vi "OFDM_SuperpositionedBitDetect.vi"(0 "Input symbols":cdb[](array[numeric]) format="%.2f", 1 "Modulation type":enum16{"QPSK(4QAM)", "64QAM", "16QAM", "BPSK"}(ring), 3 "error in (no error)":errorcluster) -> (5 "Base Bits":i8[](array[numeric]), 7 "SC Bits":i8[](array[numeric]), 10 "error out":errorcluster)   [LabVIEW 2022 SP3]
uses:
  <vilib>/addons/Modulation/Digital/General/MT Map QAM Symbols to Bits.vi
  <vilib>/addons/Modulation/Digital/General/MT Map Bits to QAM Symbols.vi
  <vilib>/addons/Modulation/Digital/General/MT Map PSK Symbols to Bits.vi
  <vilib>/addons/Modulation/Digital/General/MT Map Bits to PSK Symbols.vi
  <vilib>/addons/Modulation/niDMT.lvlib
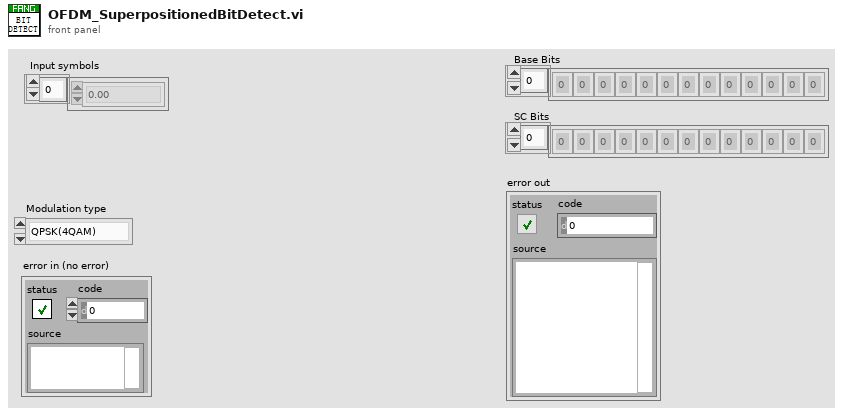
[diagram p1: front panel]
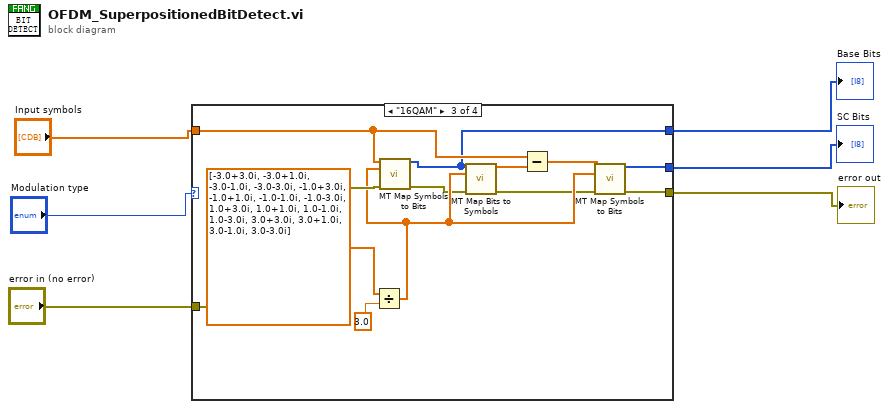
[diagram p0: block diagram]
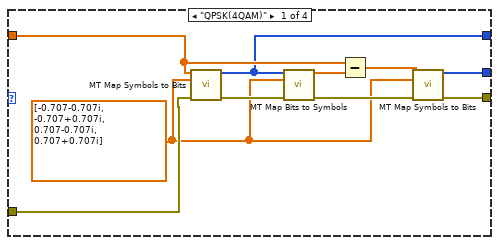
[diagram p2: hidden frame]
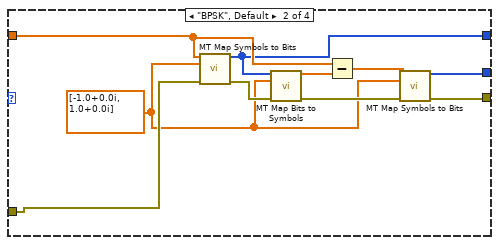
[diagram p3: hidden frame]
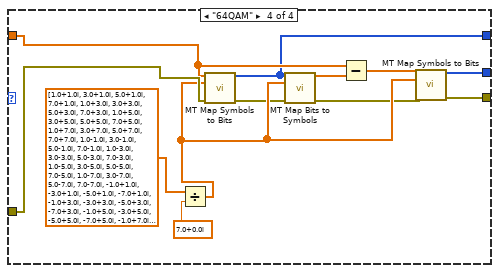
[diagram p4: hidden frame]
diagram:
  n1 = case shown="\"16QAM\"" "Modulation type" {
    tunnel: "Input symbols" -> [w13 w18 w30 w45]
    tunnel: "error in (no error)" -> [w16 w26 w38 w48]
    tunnel: [w8 w22 w35 w43] -> w3
    tunnel: [w11 w23 w34 w42] -> w2
    tunnel: [w7 w17 w27 w39] -> w1
    frame "QPSK(4QAM)" {
      w9 = cdb[] [-0.707-0.707i, -0.707+0.707i, 0.707-0.707i, 0.707+0.707i] ("symbol map")
      n2 = call-poly <vilib>:"MT Map Symbols to Bits.vi"("symbols"=w13, "symbol map"=w9, "error in (no error)"=w16) -> ("output bit stream"=w7:i8[], "error out"=w15:errorcluster)  [unwired: 11 in]
      n3 = call-poly <vilib>:"MT Map Bits to Symbols.vi"("input bit stream"=w7, "symbol map"=w9, "error in (no error)"=w15) -> ("symbols"=w14:cdb[], "error out"=w12:errorcluster)  [unwired: 11 in]
      n4 = Subtract(x=w13, y=w14) -> (x-y=w10:cdb[])
      n5 = call-poly <vilib>:"MT Map Symbols to Bits.vi"("symbols"=w10, "symbol map"=w9, "error in (no error)"=w12) -> ("output bit stream"=w8:i8[], "error out"=w11:errorcluster)  [unwired: 11 in]
    }
    frame "BPSK", Default {
      w20 = cdb[] [-1.0+0.0i, 1.0+0.0i] ("symbol map")
      n6 = call-poly <vilib>:"MT Map Symbols to Bits.vi"("symbols"=w18, "symbol map"=w20, "error in (no error)"=w26) -> ("output bit stream"=w17:i8[], "error out"=w25:errorcluster)  [unwired: 11 in]
      n7 = call-poly <vilib>:"MT Map Bits to Symbols.vi"("input bit stream"=w17, "symbol map"=w20, "error in (no error)"=w25) -> ("symbols"=w19:cdb[], "error out"=w24:errorcluster)  [unwired: 11 in]
      n8 = Subtract(x=w18, y=w19) -> (x-y=w21:cdb[])
      n9 = call-poly <vilib>:"MT Map Symbols to Bits.vi"("symbols"=w21, "symbol map"=w20, "error in (no error)"=w24) -> ("output bit stream"=w22:i8[], "error out"=w23:errorcluster)  [unwired: 11 in]
    }
    frame "16QAM" {
      n10 = Divide(x=cdb[] [-3.0+3.0i, -3.0+1.0i, -3.0-1.0i, -3.0-3.0i, -1.0+3.0i, -1.0+1.0i, -1.0-1.0i, -1.0-3.0i, 1.0+3.0i, 1.0+1.0i, 1.0-1.0i, 1.0-3.0i, 3.0+3.0i, 3.0+1.0i, 3.0-1.0i, 3.0-3.0i] ("symbol map"), y=3.0) -> (x/y=w32:cdb[])
      n11 = call-poly <vilib>:"MT Map Symbols to Bits.vi"("symbols"=w30, "symbol map"=w32, "error in (no error)"=w38) -> ("output bit stream"=w27:i8[], "error out"=w29:errorcluster)  [unwired: 11 in]
      n12 = call-poly <vilib>:"MT Map Bits to Symbols.vi"("input bit stream"=w27, "symbol map"=w32, "error in (no error)"=w29) -> ("symbols"=w31:cdb[], "error out"=w28:errorcluster)  [unwired: 11 in]
      n13 = Subtract(x=w30, y=w31) -> (x-y=w33:cdb[])
      n14 = call-poly <vilib>:"MT Map Symbols to Bits.vi"("symbols"=w33, "symbol map"=w32, "error in (no error)"=w28) -> ("output bit stream"=w35:i8[], "error out"=w34:errorcluster)  [unwired: 11 in]
    }
    frame "64QAM" {
      n15 = Divide(x=cdb[] [1.0+1.0i, 3.0+1.0i, 5.0+1.0i, 7.0+1.0i, 1.0+3.0i, 3.0+3.0i, 5.0+3.0i, 7.0+3.0i, 1.0+5.0i, 3.0+5.0i, 5.0+5.0i, 7.0+5.0i, 1.0+7.0i, 3.0+7.0i, 5.0+7.0i, 7.0+7.0i, 1.0-1.0i, 3.0-1.0i, 5.0-1.0i, 7.0-1.0i, 1.0-3.0i, 3.0-3.0i, 5.0-3.0i, 7.0-3.0i, 1.0-5.0i, 3.0-5.0i, 5.0-5.0i, 7.0-5.0i, 1.0-7.0i, 3.0-7.0i, 5.0-7.0i, 7.0-7.0i, -1.0+1.0i, -3.0+1.0i, -5.0+1.0i, -7.0+1.0i, -1.0+3.0i, -3.0+3.0i, -5.0+3.0i, -7.0+3.0i, -1.0+5.0i, -3.0+5.0i, -5.0+5.0i, -7.0+5.0i, -1.0+7.0i, -3.0+7.0i, -5.0+7.0i, -7.0+7.0i, -1.0-1.0i, -3.0-1.0i, -5.0-1.0i, -7.0-1.0i, -1.0-3.0i, -3.0-3.0i, -5.0-3.0i, -7.0-3.0i, -1.0-5.0i, -3.0-5.0i, -5.0-5.0i, -7.0-5.0i, -1.0-7.0i, -3.0-7.0i, -5.0-7.0i, -7.0-7.0i] ("appended array"), y=cdb 7.0+0.0i) -> (x/y=w47:cdb[])
      n16 = call-poly <vilib>:"MT Map Symbols to Bits.vi"("symbols"=w45, "symbol map"=w47, "error in (no error)"=w48) -> ("output bit stream"=w39:i8[], "error out"=w41:errorcluster)  [unwired: 11 in]
      n17 = call-poly <vilib>:"MT Map Bits to Symbols.vi"("input bit stream"=w39, "symbol map"=w47, "error in (no error)"=w41) -> ("symbols"=w46:cdb[], "error out"=w40:errorcluster)  [unwired: 11 in]
      n18 = Subtract(x=w45, y=w46) -> (x-y=w44:cdb[])
      n19 = call-poly <vilib>:"MT Map Symbols to Bits.vi"("symbols"=w44, "symbol map"=w47, "error in (no error)"=w40) -> ("output bit stream"=w43:i8[], "error out"=w42:errorcluster)  [unwired: 11 in]
    }
  }
  "SC Bits" <- w3
  "error out" <- w2
  "Base Bits" <- w1
